vi "Test Quaternion and Roll-Pitch-Yaw.vi"(11 "Test Case In":refnum<class "03_AR.lvclass">) -> (0 "error out":errorcluster, 3 "Test Case Out":refnum<class "03_AR.lvclass">)   [LabVIEW 2020, in "test.lvlib" / "03_AR.lvclass"]
uses:
  03_AR.lvclass
  C:/Program Files (x86)/National Instruments/LabVIEW 2020/vi.lib/Astemes/LUnit/Test Case.lvclass
  ar/Roll-Pitch-Yaw.ctl
  <vilib>/Astemes/LUnit/Test Case.lvclass/Test Case.ctl
  4993e8ee-a06a-463a-9684-69129f64d5ce.vi
  <vilib>/Astemes/LUnit/Core/LUnit Test Case/Private/Append Pass Result.vi
  <vilib>/Astemes/LUnit/Core/LUnit Test Case/Private/Append Fail Result.vi
  4993e8ee-a06a-463a-9684-69129f64d5ce.vi/9c5d11cd-9439-4240-a1ee-d9baace9c924.vi
  <vilib>/Astemes/LUnit/Core/LUnit Test Case/Private/Run In UI.vi
  <vilib>/Utility/error.llb/Clear Errors.vi
  <vilib>/Utility/error.llb/Error Cluster From Error Code.vi
  03_AR.lvclass/03_AR.ctl
  ar/ar.lvlib
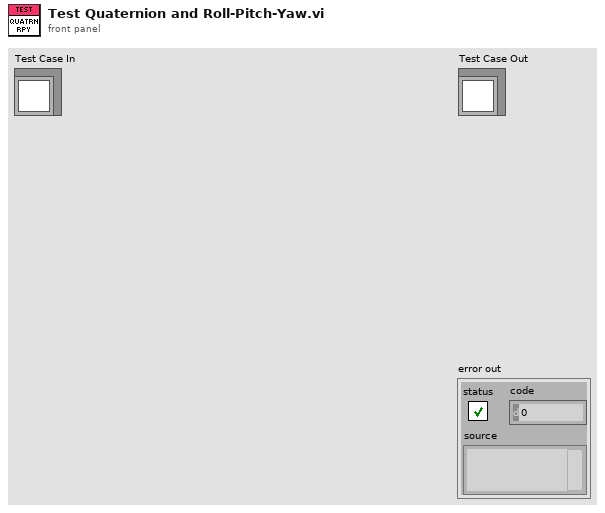
[diagram p1: front panel]
types:
  T1 = typedef "ar.lvlib/Roll-Pitch-Yaw.ctl" = cluster{"roll":dbl, "pitch":dbl, "yaw":dbl}
  T2 = typedef "ar.lvlib/Quaternion.ctl" = cluster{"w":dbl, "x":dbl, "y":dbl, "z":dbl}
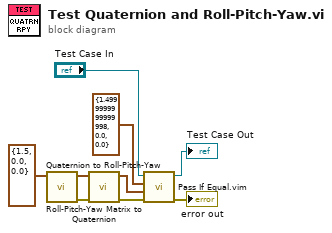
[diagram p0: block diagram]
diagram:
  n1 = call "Roll-Pitch-Yaw Matrix to Quaternion.vi"("Roll-Pitch-Yaw (rad)"=T1 {"roll"=1.5, "pitch"=0.0, "yaw"=0.0}) -> ("error out"=w6:errorcluster, "Quaternion"=w4:T2)  [unwired: 9 in]
  n2 = call "Quaternion to Roll-Pitch-Yaw.vi"("error in (no error)"=w6, "Quaternion"=w4) -> ("error out"=w2:errorcluster, "Roll-Pitch-Yaw (rad)"=w3:T1)  [unwired: 8 in]
  n3 = call "Pass If Equal.vim"("error in (no error)"=w2, "Actual"=w3, "Expected"=T1 {"roll"=1.4999999999999998, "pitch"=0.0, "yaw"=0.0} ("Roll-Pitch-Yaw (rad)"), "LUnit Test Case In"="Test Case In") -> ("error out"=→"error out":errorcluster, "LUnit Test Case Out"=→"Test Case Out":refnum<class "03_AR.lvclass">)  [unwired: 6 in]
